vi "Requests.vi"(8 "error in (no error)":errorcluster, 9 "write enable":bool=TRUE, 11 "ICPCON ET-7018 in":refnum<class "ICPCON ET-7018.lvclass">) -> (0 "error out":errorcluster, 3 "ICPCON ET-7018 out":refnum<class "ICPCON ET-7018.lvclass">)   [LabVIEW 2021, in "ICPCON ET-7018.lvclass"]
uses:
  ICPCON ET-7018.lvclass
  D:/my_projects/projects/Algorithms/Labview/21/Modbus_v121c/Network Protocol/MB/Modbus Master CR.lvclass
  D:/my_projects/projects/Algorithms/Labview/21/Modbus_v121c/Network Protocol/Network Master/Network Master.lvclass
  MB/Modbus Master CR.lvclass/Modbus Master CR.ctl
  Modbus Data Unit/Modbus Data Unit.lvclass/Modbus Data Unit.ctl
  Network Master/Network Master.lvclass/Network Master.ctl
  Master Function Definition/Read Input Registers Request.vi
  Master Function Definition/Read Input Registers Response.vi
  Network Master/Read write Master.vi
  Master Function Definition/Read Coils Request.vi
  Master Function Definition/Read Coils Response.vi
  Master Function Definition/Write Multiple Coils Request.vi
  Master Function Definition/Function data mismatch error.vi
  Master Function Definition/Write Multiple Coils Response.vi
  Modbus Data Unit/Construct PDU.vi
  Utility/Bytes to U16s.vi
  Master Function Definition/Function code mismatch error.vi
  Data Model/Error Generator.vi
  Modbus Data Unit/Deconstruct PDU.vi
  Utility/Bytes to Bits.vi
  Utility/Bits to Bytes.vi
  Modbus Data Unit/Modbus Data Unit.lvclass
  Data Model/Device Data Model.lvclass
  Transmission Data Unit/Transmission Data Unit.lvclass
  MB/Modbus Master CR.lvclass
  Network Master/Network Master.lvclass
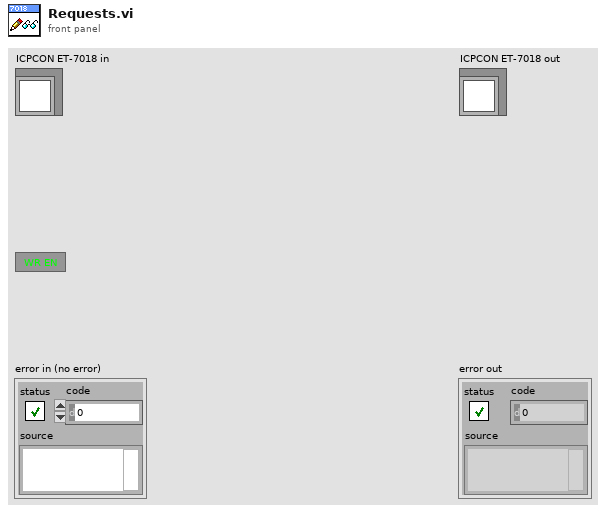
[diagram p1: front panel]
types:
  T1 = typedef "Modbus Master CR.lvclass/N channel.ctl" = cluster{"N DI channel":u16, "N DO channel":u16, "N AI channel":u16, "N AO channel":u16}
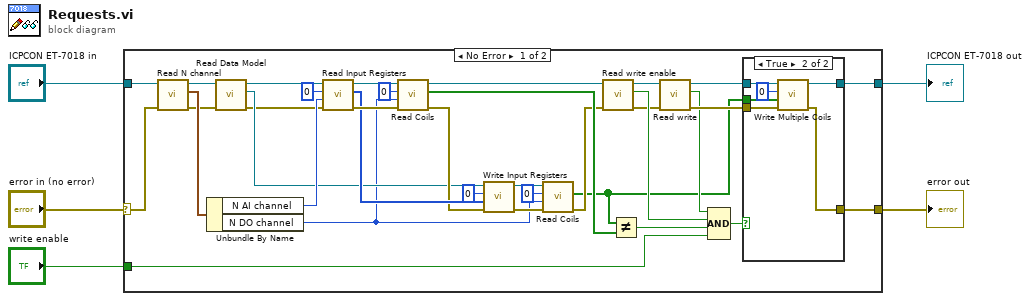
[diagram p0: block diagram]
diagram:
  n1 = case shown="No Error" "error in (no error)" {
    selector: "error in (no error)" -> [w26 w50]
    tunnel: [w39 w50] -> w3
    tunnel: [w7 w49] -> w4
    tunnel: "ICPCON ET-7018 in" -> [w28 w49]
    tunnel: "write enable" -> [w21 _]
    frame No Error {
      n2 = call "Read N channel.vi"("error in (no error)"=w26, "MB_v2 in"=w28) -> ("error out"=w25:errorcluster, "N channel"=w31:T1, "MB_v2 out"=w27:refnum<class "ICPCON ET-7018.lvclass">)  [unwired: 7 in]
      n3 = Unbundle By Name(w31) -> ("N AI channel"=w30:u16, "N DO channel"=w14:u16)
      n4 = call "Read Data Model.vi"("error in (no error)"=w25, "MB_TCP in"=w27) -> ("error out"=w10:errorcluster, "Data Model"=w24:refnum<class "Device Data Model.lvclass">, "MB_TCP out"=w11:refnum<class "ICPCON ET-7018.lvclass">)  [unwired: 7 in]
      n5 = call "Read Input Registers.vi"("error in (no error)"=w10, "number of input registers"=w30, "starting address"=u16 0, "Modbus master in"=w11) -> ("error out"=w36:errorcluster, "register values"=w33:u16[], "Modbus master out"=w37:refnum<class "ICPCON ET-7018.lvclass">)  [unwired: 5 in]
      n6 = call "Read Coils.vi"("error in (no error)"=w36, "number of coils"=w14, "starting address"=u16 0, "Modbus master in"=w37) -> ("error out"=w29:errorcluster, "coil values"=w34:bool[], "Modbus master out"=w9:refnum<class "ICPCON ET-7018.lvclass">)  [unwired: 5 in]
      n7 = call-dynamic "Write Input Registers.vi"("error in (no error)"=w29, "register values"=w33, "starting address"=u16 0, "Device Data Model in"=w24) -> ("error out"=w16:errorcluster, "Device Data Model out"=w15:refnum<class "Device Data Model.lvclass">)  [unwired: 6 in]
      n8 = call-dynamic "Read Coils.vi"("error in"=w16, "number of coils"=w14, "starting address"=u16 0, "device data model in"=w15) -> ("error out"=w12:errorcluster, "data"=w6:bool[])  [unwired: 5 in, 1 out]
      n9 = call "Read write enable.vi"("error in (no error)"=w12, "MB in"=w9) -> ("error out"=w19:errorcluster, "write enable"=w22:bool, "MB out"=w20:refnum<class "ICPCON ET-7018.lvclass">)  [unwired: 7 in]
      n10 = Not Equal?(x=w6, y=w34) -> (x != y?=w23:bool)
      n11 = call "Read write.vi"("error in (no error)"=w19, "MB in"=w20) -> ("error out"=w18:errorcluster, "Write"=w17:bool, "MB out"=w8:refnum<class "ICPCON ET-7018.lvclass">)  [unwired: 7 in]
      n12 = Compound Arithmetic op=AND(w17, w22, w23, w21) -> (w40:bool)
      n13 = case shown="True" w40 {
        tunnel: w18 -> [w42 w46]
        tunnel: [w42 w44] -> w39
        tunnel: w6 -> [_ w47]
        tunnel: w8 -> [w41 w48]
        tunnel: [w41 w43] -> w7
        frame False {
        }
        frame True {
          n14 = call "Write Multiple Coils.vi"("error in (no error)"=w46, "coil values"=w47, "starting address"=u16 0, "Modbus master in"=w48) -> ("error out"=w44:errorcluster, "Modbus master out"=w43:refnum<class "ICPCON ET-7018.lvclass">)  [unwired: 6 in]
        }
      }
    }
    frame Error {
    }
  }
  "error out" <- w3
  "ICPCON ET-7018 out" <- w4
